vi "P2_calculcate.vi"(8 "Points":dbl[][](array[numeric])=[[-200.0, -0.1], [-400.0, -0.2], [-600.0, -0.5], [-800.0, -100.0]], 11 "P1i":T1) -> (3 "P2i":cluster{dbl[], dbl[]})   [LabVIEW 2015]
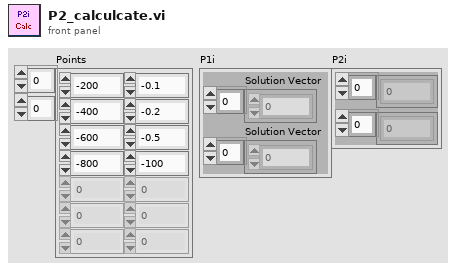
[diagram p1: front panel]
types:
  T1 = cluster{"Solution Vector":dbl[], "Solution Vector":dbl[]}
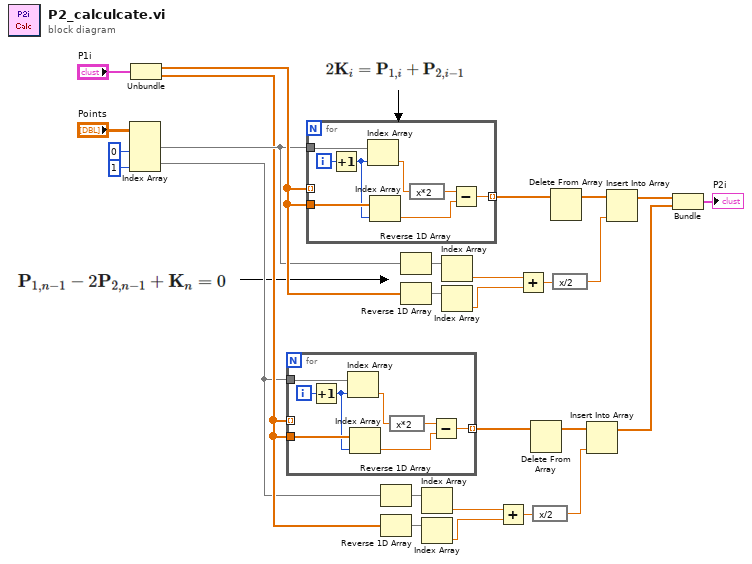
[diagram p0: block diagram]
diagram:
  n1 = Index Array(array="Points", index (col) #1=0 ("disabled index (col)"), index (col) #2=1 ("index (col)")) -> (element #1=w14:dbl[], element #2=w4:dbl[])  [unwired: 2 in]
  n2 = Unbundle("P1i") -> ("Solution Vector"=w15:dbl[], "Solution Vector"=w5:dbl[])
  n3 = for {
    tunnel: [w34] -> w13 mode=indexing
    tunnel: w4 -> [w33]
    tunnel: w5 -> [w30]
    tunnel: w5 -> [_] mode=indexing
    i -> [w32]
    n4 = Increment(x=w32) -> (x+1=w29:i32)
    n5 = Index Array(array=w33, index=w29) -> (element=w31:dbl)
    n6 = Index Array(array=w30, index=w29) -> (element=w28:dbl)
    n7 = expression code="x*2"(w31) -> (w35:dbl)
    n8 = Subtract(x=w35, y=w28) -> (x-y=w34:dbl)
  }
  n9 = for {
    tunnel: [w42] -> w20 mode=indexing
    tunnel: w14 -> [w41]
    tunnel: w15 -> [w38]
    tunnel: w15 -> [_] mode=indexing
    i -> [w40]
    n10 = Increment(x=w40) -> (x+1=w37:i32)
    n11 = Index Array(array=w41, index=w37) -> (element=w39:dbl)
    n12 = Index Array(array=w38, index=w37) -> (element=w36:dbl)
    n13 = expression code="x*2"(w39) -> (w43:dbl)
    n14 = Subtract(x=w43, y=w36) -> (x-y=w42:dbl)
  }
  n15 = Reverse 1D Array(array=w4) -> (reversed array=w6:dbl[])
  n16 = Reverse 1D Array(array=w5) -> (reversed array=w7:dbl[])
  n17 = Reverse 1D Array(array=w14) -> (reversed array=w27:dbl[])
  n18 = Reverse 1D Array(array=w15) -> (reversed array=w26:dbl[])
  n19 = Index Array(array=w6) -> (element=w8:dbl)  [unwired: 1 in]
  n20 = Index Array(array=w7) -> (element=w9:dbl)  [unwired: 1 in]
  n21 = Index Array(array=w27) -> (element=w25:dbl)  [unwired: 1 in]
  n22 = Index Array(array=w26) -> (element=w24:dbl)  [unwired: 1 in]
  n23 = Add(x=w8, y=w9) -> (x+y=w10:dbl)
  n24 = Add(x=w25, y=w24) -> (x+y=w23:dbl)
  n25 = Delete From Array(array=w13) -> (array with subset deleted=w11:dbl[])  [unwired: 2 in, 1 out]
  n26 = expression code="x/2"(w10) -> (w12:dbl)
  n27 = Delete From Array(array=w20) -> (array with subset deleted=w22:dbl[])  [unwired: 2 in, 1 out]
  n28 = expression code="x/2"(w23) -> (w21:dbl)
  n29 = Insert Into Array(array=w11, new element=w12) -> (w2:dbl[])  [unwired: 1 in]
  n30 = Insert Into Array(array=w22, new element=w21) -> (w3:dbl[])  [unwired: 1 in]
  n31 = Bundle(w3, w2) -> (→"P2i":cluster{dbl[], dbl[]})  [unwired: 1 in]
